vi "ASIC_WRITE THX THX3 READ ADC muy simple.vi"(0 "ftHandle_in":u32, 1 "Sumador":u8, 2 "THX":u16, 3 "THX+3":u16, 5 "error in":errorcluster, 8 "Espera acceso USB 2":u32) -> (14 "ftHandle_out":u32, 16 "HLTHx":dbl, 17 "LLTHx":dbl, 19 "error out":errorcluster)   [LabVIEW 2019]
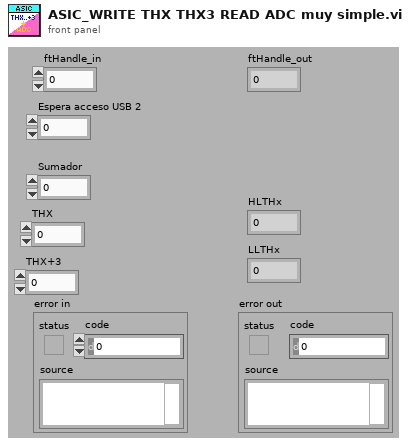
[diagram p1: front panel]
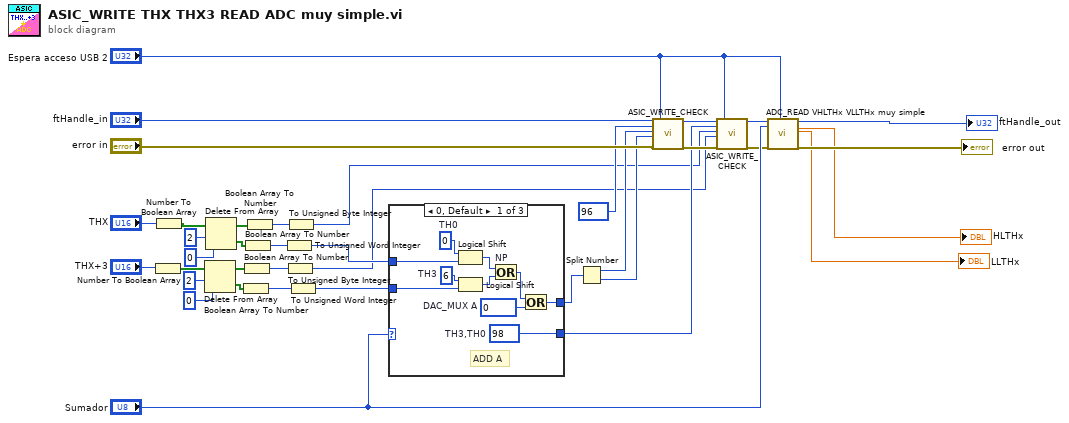
[diagram p0: block diagram]
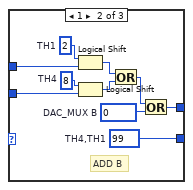
[diagram p2: hidden frame]
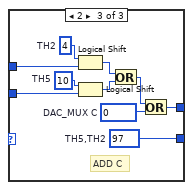
[diagram p3: hidden frame]
diagram:
  n1 = Number To Boolean Array(number="THX+3") -> (Boolean array=w15:bool[])
  n2 = Number To Boolean Array(number="THX") -> (Boolean array=w20:bool[])
  n3 = Delete From Array(array=w15, length=2, index=0) -> (deleted portion=w24:bool[], array with subset deleted=w23:bool[])
  n4 = Delete From Array(array=w20, length=2, index=0) -> (deleted portion=w22:bool[], array with subset deleted=w21:bool[])
  n5 = Boolean Array To Number(Boolean array=w24) -> (number=w26:u32)
  n6 = Boolean Array To Number(Boolean array=w23) -> (number=w28:u32)
  n7 = Boolean Array To Number(Boolean array=w22) -> (number=w25:u32)
  n8 = Boolean Array To Number(Boolean array=w21) -> (number=w27:u32)
  n9 = To Unsigned Word Integer(number=w25) -> (unsigned 16bit integer=w36:u16)
  n10 = To Unsigned Byte Integer(number=w28) -> (unsigned 8bit integer=w3:u8)
  n11 = To Unsigned Byte Integer(number=w27) -> (unsigned 8bit integer=w4:u8)
  n12 = To Unsigned Word Integer(number=w26) -> (unsigned 16bit integer=w37:u16)
  n13 = case shown="0, Default" "Sumador" {
    tunnel: [w47 w57 w67] -> w5
    tunnel: w36 -> [w46 w56 w66]
    tunnel: w37 -> [w45 w55 w65]
    tunnel: [w39 w49 w59] -> w8
    frame 0, Default {
      w38 = u16 0  # DAC_MUX A
      w43 = i8 6  # TH3
      w44 = i8 0  # TH0
      w47 = u8 98  # TH3,TH0
      # "ADD A"
      n14 = Logical Shift(y=w44, x=w46) -> (x << y=w41:u16)
      n15 = Logical Shift(y=w43, x=w45) -> (x << y=w42:u16)
      n16 = Or "NP"(x=w41, y=w42) -> (x .or. y?=w40:u16)
      n17 = Or(x=w40, y=w38) -> (x .or. y?=w39:u16)
    }
    frame 1 {
      w48 = u16 0  # DAC_MUX B
      w53 = i8 8  # TH4
      w54 = i8 2  # TH1
      w57 = u8 99  # TH4,TH1
      # "ADD B"
      n18 = Logical Shift(y=w54, x=w56) -> (x << y=w51:u16)
      n19 = Logical Shift(y=w53, x=w55) -> (x << y=w52:u16)
      n20 = Or(x=w51, y=w52) -> (x .or. y?=w50:u16)
      n21 = Or(x=w50, y=w48) -> (x .or. y?=w49:u16)
    }
    frame 2 {
      w58 = u16 0  # DAC_MUX C
      w63 = i8 10  # TH5
      w64 = i8 4  # TH2
      w67 = u8 97  # TH5,TH2
      # "ADD C"
      n22 = Logical Shift(y=w64, x=w66) -> (x << y=w61:u16)
      n23 = Logical Shift(y=w63, x=w65) -> (x << y=w62:u16)
      n24 = Or(x=w61, y=w62) -> (x .or. y?=w60:u16)
      n25 = Or(x=w60, y=w58) -> (x .or. y?=w59:u16)
    }
  }
  n26 = Split Number(x=w8) -> (hi(x)=w10:u8, lo(x)=w11:u8)
  n27 = call "ASIC_WRITE_CHECK.vi"("ftHandle_in"="ftHandle_in", "Direccion Registro Asic"=u8 96, "Byte Alto"=w10, "Byte Bajo"=w11, "error in"="error in", "Espera acceso USB 2"="Espera acceso USB 2") -> ("ftHandle_out"=w6:u32, "error out"=w7:errorcluster)  [unwired: 11 in, 1 out]
  n28 = call "ASIC_WRITE_CHECK.vi"("ftHandle_in"=w6, "Direccion Registro Asic"=w5, "Byte Alto"=w4, "Byte Bajo"=w3, "error in"=w7, "Espera acceso USB 2"="Espera acceso USB 2") -> ("ftHandle_out"=w12:u32, "error out"=w13:errorcluster)  [unwired: 11 in, 1 out]
  n29 = call "ADC_READ VHLTHx VLLTHx muy simple.vi"("ftHandle_out 2"=w12, "Sumador"="Sumador", "error out 2"=w13, "Espera acceso FT"="Espera acceso USB 2") -> ("ftHandle_out"=→"ftHandle_out":u32, "HLTHx"=→"HLTHx":dbl, "LLTHx"=→"LLTHx":dbl, "error out"=→"error out":errorcluster)  [unwired: 12 in]
